vi "ConfigChecker.vi"() -> ()   [LabVIEW 2014]
panel:
  out "Output":string
  out "Should Stop?":bool
  out "Extra Lines Removed":string[](array[string])
  out "result string":string
  out "NonSensed":string[](array[string])
  in  "Auto Config File":path=path "C:/Users/Matthew/Desktop/Auto Config Testing/autoexample.txt"
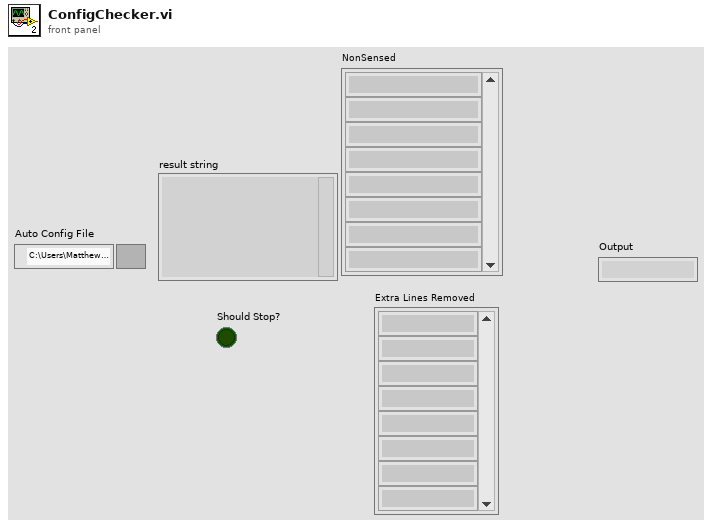
[diagram p1: front panel]
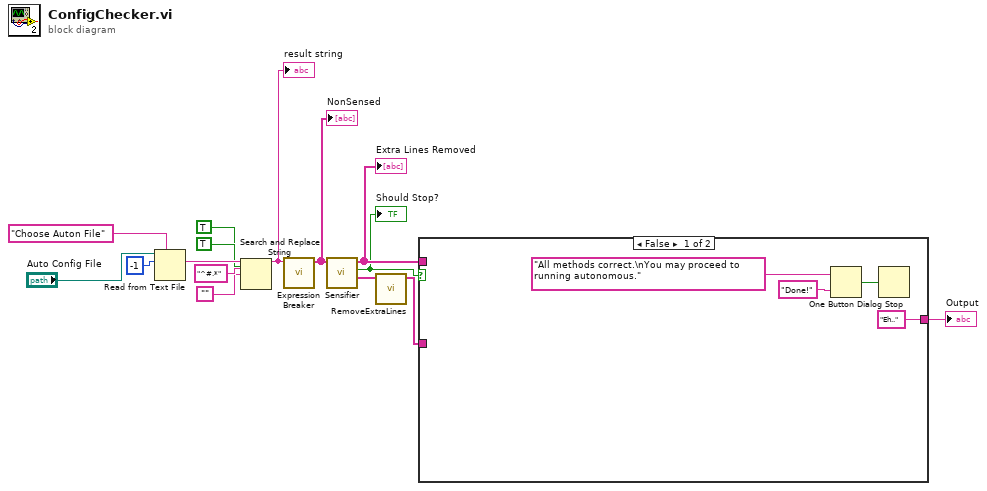
[diagram p0: block diagram]
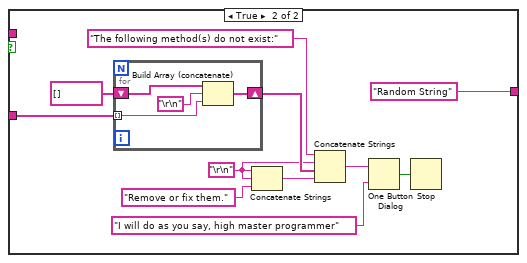
[diagram p2: hidden frame]
diagram:
  n1 = Read from Text File(prompt (Open existing file)="Choose Auton File", file (use dialog)="Auto Config File", count=-1) -> (text=w13:string)  [unwired: 1 in, 3 out]
  n2 = Search and Replace String(replace all?=TRUE ("replace all? (F)"), multiline?=TRUE ("multiline? (F)"), input string=w13, search string="^#.*" ("regular expression"), replace string="") -> (result string=w8:string)  [unwired: 3 in, 3 out]
  "result string" <- w8
  n3 = call "Expression Breaker.vi"("result string"=w8) -> ("Array"=w7:string[])  [unwired: 10 in]
  "NonSensed" <- w7
  n4 = call "Sensifier.vi"("Array"=w7) -> ("Removed Strings"=w6:string[], "Has Errors?"=w3:bool, "Sensed"=w4:string[])  [unwired: 8 in]
  "Extra Lines Removed" <- w4
  "Should Stop?" <- w3
  n5 = call "RemoveExtraLines.vi"("Sensed"=w6) -> ("Output"=w5:string[])  [unwired: 10 in]
  n6 = case shown="False" w3 {
    tunnel: w5 -> [_ w25]
    tunnel: w4 -> [_ _]
    tunnel: ["Eh.." "Random String"] -> w1
    frame False {
      n7 = One Button Dialog(message="All methods correct.\nYou may proceed to running autonomous.", button name ("OK")="Done!") -> (true=w19:bool)
      n8 = Stop(stop? (T)=w19) -> ()
    }
    frame True {
      w22 = "\r\n"
      n9 = for {
        shift-right: [w34] -> w30
        shift-left: string[] [] -> [w31]
        tunnel: w25 -> [w33] mode=indexing
        n10 = Build Array (concatenate)(w31, "\r\n", w33) -> (w34:string[])
      }
      n11 = Concatenate Strings(w22, w22, "Remove or fix them.") -> (w26:string)
      n12 = Concatenate Strings("The following method(s) do not exist:", w22, w30, w26) -> (w29:string)
      n13 = One Button Dialog(message=w29, button name ("OK")="I will do as you say, high master programmer") -> (true=w28:bool)
      n14 = Stop(stop? (T)=w28) -> ()
    }
  }
  "Output" <- w1
